vi "Disconnect.vi"(8 "error in (no error)":errorcluster) -> (0 "error out":errorcluster, 3 "Feedback":string)   [LabVIEW 2017]
doc: "Disconnects the specified interface from a wireless network."
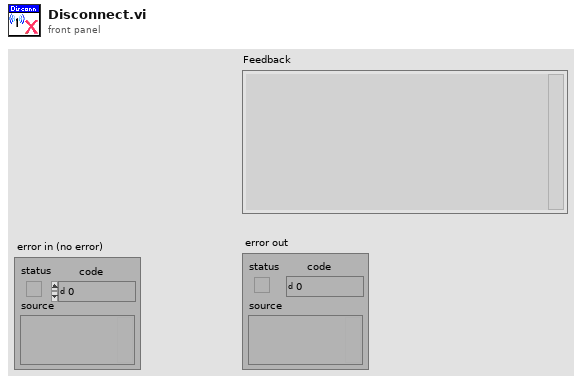
[diagram p1: front panel]
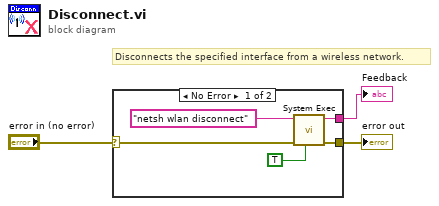
[diagram p0: block diagram]
diagram:
  # "Disconnects the specified interface from a wireless network."
  n1 = case shown="No Error" "error in (no error)" {
    selector: "error in (no error)" -> [w6 w9]
    tunnel: [w5 w9] -> w2
    tunnel: [w4 _] -> w1
    frame No Error {
      n2 = call <vilib>:"System Exec.vi"("run minimized? (F)"=TRUE, "error in (no error)"=w6, "command line"="netsh wlan disconnect") -> ("error out"=w5:errorcluster, "standard output"=w4:string)  [unwired: 5 in, 2 out]
    }
    frame Error {
    }
  }
  "error out" <- w2
  "Feedback" <- w1
